vi "gfitsio-movnam-hdu.vi"(7 "extname":string, 8 "error in (no error)":errorcluster, 9 "extver (0:ignore extver)":i32, 10 "hdutype (ANY_HDU)":T2=-1 items=["ANY_HDU"=-1, "IMAGE_HDU"=0, "ASCII_TBL"=1, "BINARY_TBL"=2], 11 "gfits refnum":T1) -> (0 "error out":errorcluster, 3 "dup gfits refnum":T1)   [LabVIEW 2019, in "gfitsio.lvlib"]
doc: "Moves to the (first) HDU which has the specified extension type and EXTNAME and EXTVER keyword values (or HDUNAME and HDUVER keywords). The hdutype parameter may have a value of IMAGE_HDU, ASCII_TBL, BINARY_TBL, or ANY_HDU where ANY_HDU means that only the extname and extver values will be used to locate the correct extension. If the input value of extver is 0 then the EXTVER keyword is ignored and the first HDU with a matching EXTNAME (or HDUNAME) keyword will be found. If no matching HDU is found in the file then the current HDU will remain unchanged and an error will be returned."
uses:
  gfitsio.lvlib
  cfitsio-hdutypes.ctl
  gfitsio-refnum.ctl
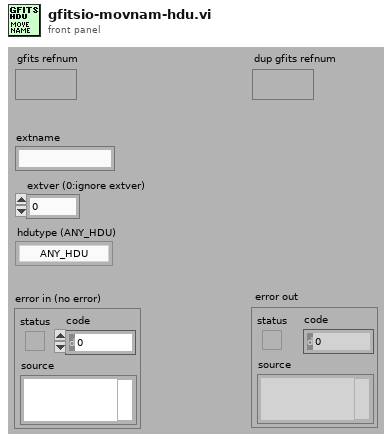
[diagram p1: front panel]
types:
  T1 = typedef "gfitsio.lvlib/gfitsio-refnum.ctl" = refnum<k1>
  T2 = typedef "gfitsio.lvlib/cfitsio-hdutypes.ctl" = i32
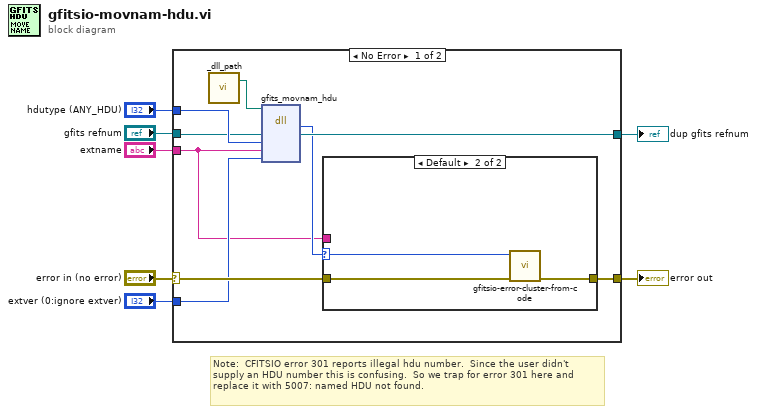
[diagram p0: block diagram]
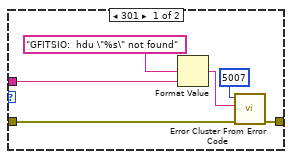
[diagram p2: hidden frame]
diagram:
  # "Note:  CFITSIO error 301 reports illegal hdu number.  Since the user didn't supply an HDU number this is confusing.  So we trap for error 301 here and replace it with 5007: named HDU not found."
  n1 = case shown="No Error" "error in (no error)" {
    selector: "error in (no error)" -> [w16 w27]
    tunnel: [w15 w27] -> w6
    tunnel: "extname" -> [w9 _]
    tunnel: "extver (0:ignore extver)" -> [w14 _]
    tunnel: "hdutype (ANY_HDU)" -> [w13 _]
    tunnel: [w11 w26] -> w2
    tunnel: "gfits refnum" -> [w12 w26]
    frame No Error {
      n2 = call "_dll_path.vi"() -> ("Path"=w8:path)  [unwired: 1 in]
      n3 = dll-call lib="?" fn="gfits_movnam_hdu"(path in=w8, "refnum"=w12, "hdutype"=w13, "extname"=w9, "extver"=w14) -> ("return type"=w10:i32, "refnum"=w11:T1)  [unwired: 4 in, 3 out]
      n4 = case shown="Default" w10 {
        selector: w10 -> [_ w23]
        tunnel: w16 -> [w21 w25]
        tunnel: [w22 w24] -> w15
        tunnel: w9 -> [w18 _]
        frame 301 {
          n5 = Format Value(format string="GFITSIO:  hdu \"%s\" not found", value (0)=w18) -> (output string=w20:string)  [unwired: 1 out]
          n6 = call <vilib>:"Error Cluster From Error Code.vi"("error in (no error)"=w21, "error message (\"\")"=w20, "error code (0)"=5007) -> ("error out"=w22:errorcluster)  [unwired: 1 in, 5 out]
        }
        frame Default {
          n7 = call "gfitsio-error-cluster-from-code.vi"("error in (no error)"=w25, "error code"=w23) -> ("error out"=w24:errorcluster)  [unwired: 9 out]
        }
      }
    }
    frame Error {
    }
  }
  "error out" <- w6
  "dup gfits refnum" <- w2
